vi "MBFL_Controller.vi"(0 "K":dbl[](array[numeric]), 1 "q_ref":dbl[](array[numeric]), 2 "q1":dbl, 3 "q2":dbl, 4 "q3":dbl, 5 "q4":dbl, 7 "K1":dbl, 9 "K2":dbl, 11 "K3":dbl, 13 "K4":dbl) -> (16 "u_out":dbl)   [LabVIEW 2021]
uses:
  <vilib>/Analysis/baseanly.llb/Real A x B.vi
  <vilib>/Analysis/Matrix/Numeric/Conversions/Matrix To Array - RM.vi
  <vilib>/Analysis/Matrix/Numeric/Conversions/Array To Matrix - RA2.vi
  <vilib>/Analysis/Matrix/Numeric/Multiply/Multiply - RM,R.vi
  <vilib>/Analysis/Matrix/NI_Matrix.lvlib
  <vilib>/Analysis/NI_AALBase.lvlib
panel:
  out "Etta(q)":dbl(graph)
  out "q1":dbl(graph)
  out "v(q)":dbl(graph)
  out "Control input u":dbl(graph)
  out "Gamma(q)":dbl(graph)
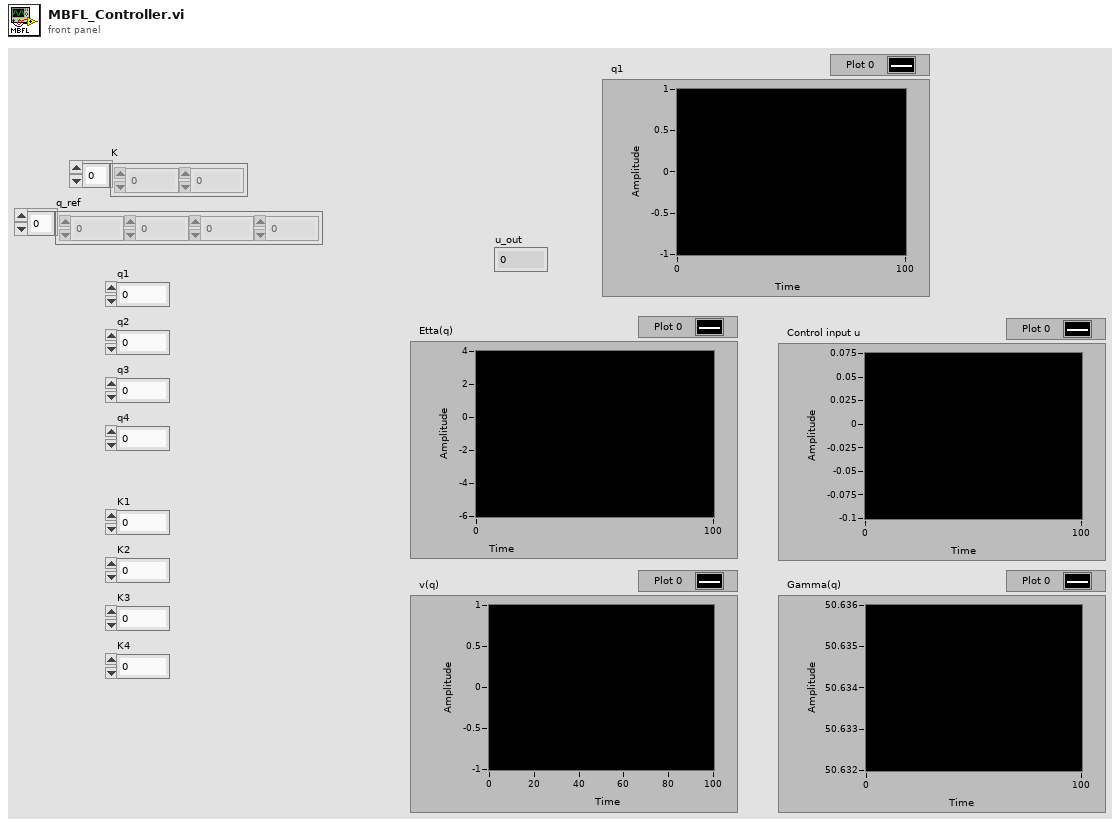
[diagram p1: front panel]
types:
  T1 = typedef "NI_Matrix.lvlib/RealMatrix.ctl" = dbl[][]
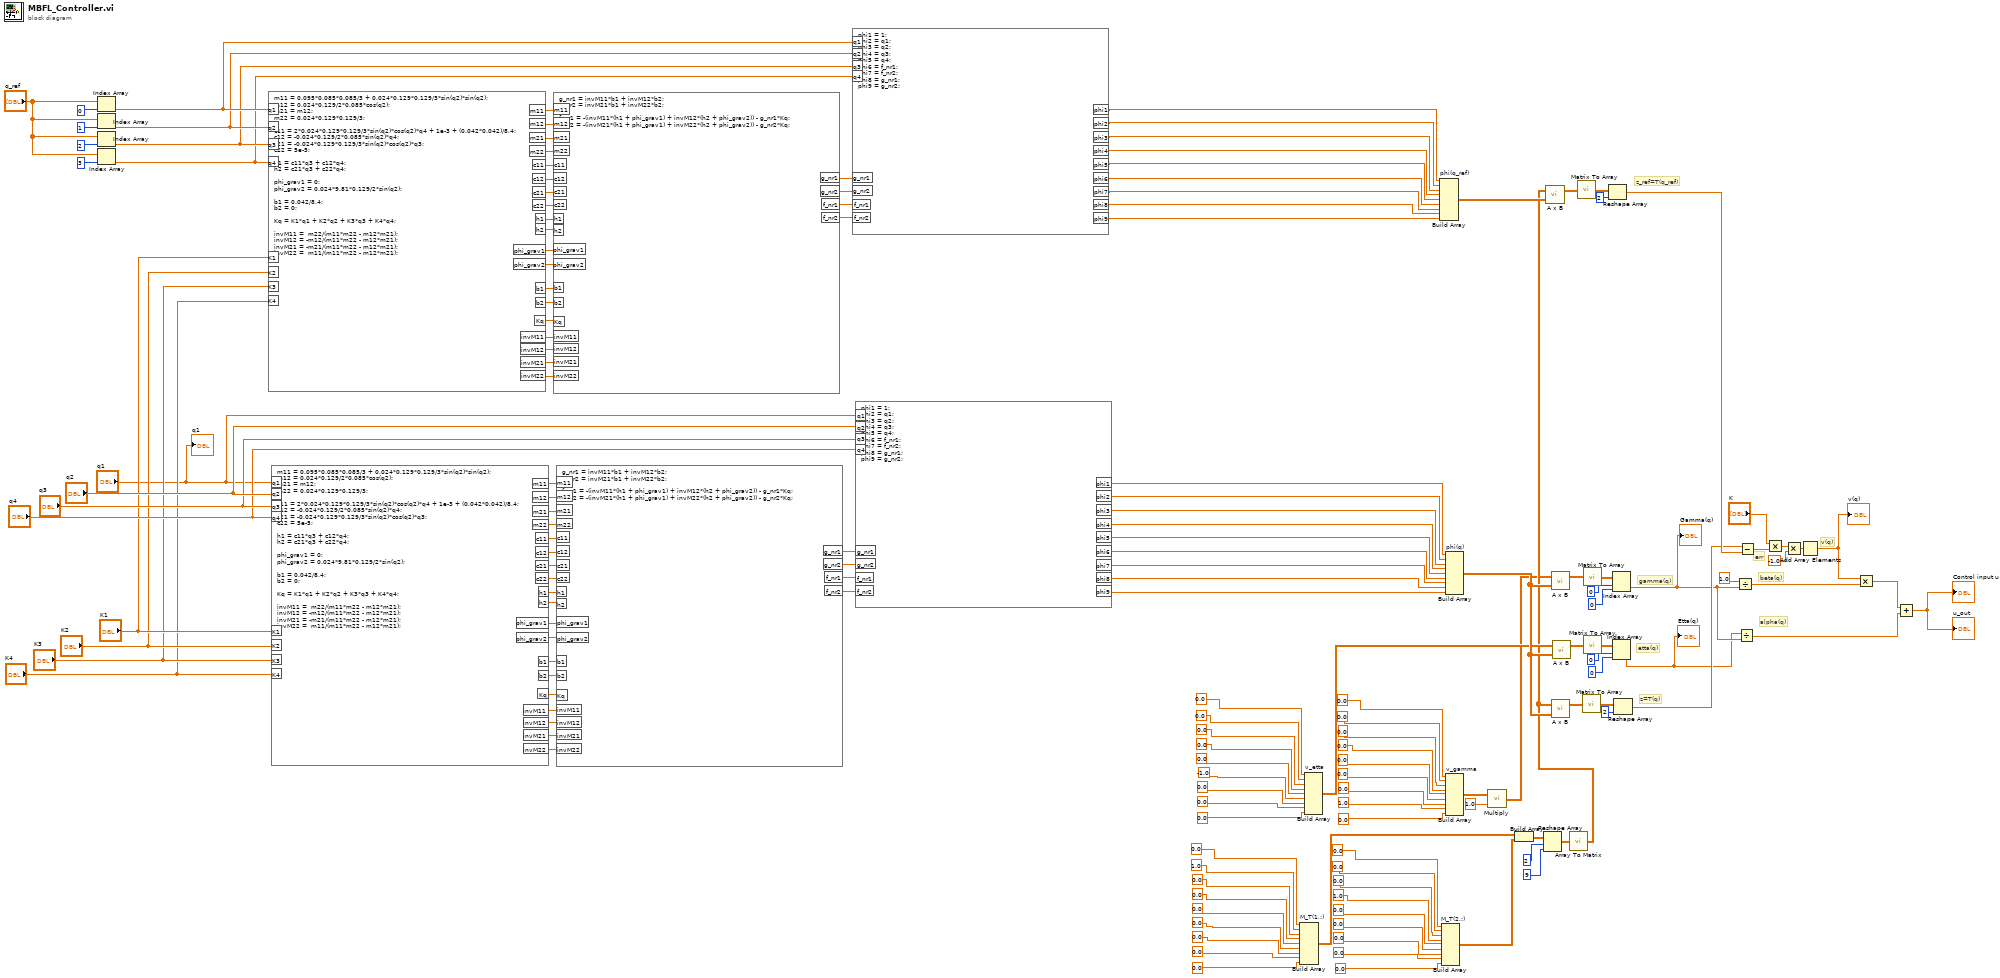
[diagram p0: block diagram]
diagram:
  # "alpha(q)"
  # "beta(q)"
  # "z_ref=T(q_ref)"
  # "v(q)"
  # "err"
  # "z=T(q)"
  # "etta(q)"
  # "gamma(q)"
  n1 = Index Array(array="q_ref", index=0 ("index 3")) -> (element=w29:dbl)
  n2 = Index Array(array="q_ref", index=1 ("index 4")) -> (element=w27:dbl)
  n3 = Index Array(array="q_ref", index=2 ("index 3")) -> (element=w26:dbl)
  n4 = Index Array(array="q_ref", index=3 ("index 4")) -> (element=w25:dbl)
  n5 = formula code="m11 = 0.095*0.085*0.085/3 + 0.024*0.129*0.129/3*sin(q2)*sin(q2);\nm12 = 0.024*0.129/2*0.085*cos(q2);\nm21 = m12;\nm22 = 0.024*0.129*0.129/3;\n\nc11 = 2*0.024*0.129*0.129/3*sin(q2)*cos(q2)*q4 + 1e-3 + (0.042*0.042)/8.4;\nc12 = -0.024*0.129/2*0.085*sin(q2)*q4;\nc21 = -0.024*0.129*0.129/3*sin(q2)*cos(q2)*q3;\nc22 = 5e-5;\n\nh1 = c11*q3 + c12*q4;\nh2 = c21*q3 + c22*q4;\n\nphi_grav1 = 0;\nphi_grav2 = 0.024*9.81*0.129/2*sin(q2);\n\nb1 = 0.042/8.4;\nb2 = 0;\n\nKq = K1*q1 + K2*q2 + K3*q3 + K4*q4;\n\ninvM11 =  m22/(m11*m22 - m12*m21);\ninvM12 = -m12/(m11*m22 - m12*m21);\ninvM21 = -m21/(m11*m22 - m12*m21);\ninvM22 =  m11/(m11*m22 - m12*m21);"("q1"=w29, "q2"=w27, "q3"=w26, "q4"=w25, "K1"="K1", "K2"="K2", "K3"="K3", "K4"="K4") -> ("m11"=w70:dbl, "m12"=w69:dbl, "m21"=w68:dbl, "m22"=w67:dbl, "c11"=w66:dbl, "c12"=w65:dbl, "c21"=w64:dbl, "c22"=w63:dbl, "h1"=w62:dbl, "h2"=w61:dbl, "phi_grav1"=w60:dbl, "phi_grav2"=w59:dbl, "b1"=w58:dbl, "b2"=w57:dbl, "Kq"=w56:dbl, "invM11"=w55:dbl, "invM12"=w54:dbl, "invM21"=w53:dbl, "invM22"=w52:dbl)
  n6 = formula code="m11 = 0.095*0.085*0.085/3 + 0.024*0.129*0.129/3*sin(q2)*sin(q2);\nm12 = 0.024*0.129/2*0.085*cos(q2);\nm21 = m12;\nm22 = 0.024*0.129*0.129/3;\n\nc11 = 2*0.024*0.129*0.129/3*sin(q2)*cos(q2)*q4 + 1e-3 + (0.042*0.042)/8.4;\nc12 = -0.024*0.129/2*0.085*sin(q2)*q4;\nc21 = -0.024*0.129*0.129/3*sin(q2)*cos(q2)*q3;\nc22 = 5e-5;\n\nh1 = c11*q3 + c12*q4;\nh2 = c21*q3 + c22*q4;\n\nphi_grav1 = 0;\nphi_grav2 = 0.024*9.81*0.129/2*sin(q2);\n\nb1 = 0.042/8.4;\nb2 = 0;\n\nKq = K1*q1 + K2*q2 + K3*q3 + K4*q4;\n\ninvM11 =  m22/(m11*m22 - m12*m21);\ninvM12 = -m12/(m11*m22 - m12*m21);\ninvM21 = -m21/(m11*m22 - m12*m21);\ninvM22 =  m11/(m11*m22 - m12*m21);"("q1"="q1", "q2"="q2", "q3"="q3", "q4"="q4", "K1"="K1", "K2"="K2", "K3"="K3", "K4"="K4") -> ("m11"=w96:dbl, "m12"=w95:dbl, "m21"=w94:dbl, "m22"=w93:dbl, "c11"=w92:dbl, "c12"=w91:dbl, "c21"=w90:dbl, "c22"=w89:dbl, "h1"=w88:dbl, "h2"=w87:dbl, "phi_grav1"=w86:dbl, "phi_grav2"=w85:dbl, "b1"=w84:dbl, "b2"=w83:dbl, "Kq"=w82:dbl, "invM11"=w81:dbl, "invM12"=w80:dbl, "invM21"=w79:dbl, "invM22"=w78:dbl)
  n7 = formula code="g_nr1 = invM11*b1 + invM12*b2;\ng_nr2 = invM21*b1 + invM22*b2;\n\nf_nr1 = -(invM11*(h1 + phi_grav1) + invM12*(h2 + phi_grav2)) - g_nr1*Kq;\nf_nr2 = -(invM21*(h1 + phi_grav1) + invM22*(h2 + phi_grav2)) - g_nr2*Kq;"("m11"=w70, "m12"=w69, "m21"=w68, "m22"=w67, "invM11"=w55, "invM12"=w54, "invM21"=w53, "invM22"=w52, "c11"=w66, "c12"=w65, "c21"=w64, "c22"=w63, "h1"=w62, "h2"=w61, "phi_grav1"=w60, "phi_grav2"=w59, "b1"=w58, "b2"=w57, "Kq"=w56) -> ("g_nr1"=w51:dbl, "g_nr2"=w50:dbl, "f_nr1"=w49:dbl, "f_nr2"=w48:dbl)
  n8 = formula code="g_nr1 = invM11*b1 + invM12*b2;\ng_nr2 = invM21*b1 + invM22*b2;\n\nf_nr1 = -(invM11*(h1 + phi_grav1) + invM12*(h2 + phi_grav2)) - g_nr1*Kq;\nf_nr2 = -(invM21*(h1 + phi_grav1) + invM22*(h2 + phi_grav2)) - g_nr2*Kq;"("m11"=w96, "m12"=w95, "m21"=w94, "m22"=w93, "invM11"=w81, "invM12"=w80, "invM21"=w79, "invM22"=w78, "c11"=w92, "c12"=w91, "c21"=w90, "c22"=w89, "h1"=w88, "h2"=w87, "phi_grav1"=w86, "phi_grav2"=w85, "b1"=w84, "b2"=w83, "Kq"=w82) -> ("g_nr1"=w77:dbl, "g_nr2"=w76:dbl, "f_nr1"=w75:dbl, "f_nr2"=w74:dbl)
  n9 = formula code="phi1 = 1;\nphi2 = q1;\nphi3 = q2;\nphi4 = q3;\nphi5 = q4;\nphi6 = f_nr1;\nphi7 = f_nr2;\nphi8 = g_nr1;\nphi9 = g_nr2;"("q1"=w29, "q2"=w27, "q3"=w26, "q4"=w25, "g_nr1"=w51, "g_nr2"=w50, "f_nr1"=w49, "f_nr2"=w48) -> ("phi1"=w47:dbl, "phi2"=w46:dbl, "phi3"=w45:dbl, "phi4"=w44:dbl, "phi5"=w43:dbl, "phi6"=w42:dbl, "phi7"=w41:dbl, "phi8"=w40:dbl, "phi9"=w39:dbl)
  n10 = formula code="phi1 = 1;\nphi2 = q1;\nphi3 = q2;\nphi4 = q3;\nphi5 = q4;\nphi6 = f_nr1;\nphi7 = f_nr2;\nphi8 = g_nr1;\nphi9 = g_nr2;"("q1"="q1", "q2"="q2", "q3"="q3", "q4"="q4", "g_nr1"=w77, "g_nr2"=w76, "f_nr1"=w75, "f_nr2"=w74) -> ("phi1"=w105:dbl, "phi2"=w104:dbl, "phi3"=w103:dbl, "phi4"=w102:dbl, "phi5"=w101:dbl, "phi6"=w100:dbl, "phi7"=w99:dbl, "phi8"=w98:dbl, "phi9"=w97:dbl)
  n11 = Build Array "M_T(1,:)"(0.0, 1.0, 0.0, 0.0, 0.0, 0.0, 0.0, 0.0, 0.0) -> (w111:T1)
  n12 = Build Array "v_etta"(0.0, 0.0, 0.0, 0.0, 0.0, -1.0, 0.0, 0.0, 0.0) -> (w150:T1)
  n13 = Build Array "phi(q_ref)"(w47, w46, w45, w44, w43, w42, w41, w40, w39) -> (w35:T1)
  n14 = Build Array "M_T(2,:)"(0.0, 0.0, 0.0, 1.0, 0.0, 0.0, 0.0, 0.0, 0.0) -> (w110:T1)
  n15 = Build Array "phi(q)"(w105, w104, w103, w102, w101, w100, w99, w98, w97) -> (w151:T1)
  n16 = Build Array "v_gamma"(0.0, 0.0, 0.0, 0.0, 0.0, 0.0, 0.0, 1.0, 0.0) -> (w15:T1)
  n17 = call-poly <vilib>:"Multiply.vi"("Real Scalar c"=1.0, "Real Matrix A"=w15) -> ("A * c"=w17:T1)
  n18 = Build Array(w111, w110) -> (w109:dbl[][][])
  n19 = Reshape Array(w109, 2, 9) -> (w106:dbl[][])
  n20 = call-poly <vilib>:"A x B.vi"("B"=w151, "A"=w17) -> ("A x B"=w146:T1)  [unwired: 1 out]
  n21 = call-poly <vilib>:"A x B.vi"("B"=w151, "A"=w150) -> ("A x B"=w141:T1)  [unwired: 1 out]
  n22 = call-poly <vilib>:"Array To Matrix.vi"("Real 2D Array"=w106) -> ("Real Matrix"=w34:T1)
  n23 = call-poly <vilib>:"A x B.vi"("B"=w35, "A"=w34) -> ("A x B"=w38:T1)  [unwired: 1 out]
  n24 = call-poly <vilib>:"A x B.vi"("B"=w151, "A"=w34) -> ("A x B"=w142:T1)  [unwired: 1 out]
  n25 = call-poly <vilib>:"Matrix To Array.vi"("Real Matrix"=w38) -> ("Real 2D Array"=w37:dbl[][])
  n26 = call-poly <vilib>:"Matrix To Array.vi"("Real Matrix"=w142) -> ("Real 2D Array"=w140:dbl[][])
  n27 = call-poly <vilib>:"Matrix To Array.vi"("Real Matrix"=w146) -> ("Real 2D Array"=w149:dbl[][])
  n28 = call-poly <vilib>:"Matrix To Array.vi"("Real Matrix"=w141) -> ("Real 2D Array"=w145:dbl[][])
  n29 = Reshape Array(w37, 2 ("dimension size")) -> (w12:dbl[])
  n30 = Index Array ("Index Array 2")(array=w149, index (row)=0 ("index 3"), index (col)=0 ("index 4")) -> (element=w7:dbl)
  "Gamma(q)" <- w7
  n31 = Index Array ("Index Array 2")(array=w145, index (row)=0 ("index 3"), index (col)=0 ("index 4")) -> (element=w6:dbl)
  "Etta(q)" <- w6
  n32 = Reshape Array(w140, 2 ("dimension size")) -> (w11:dbl[])
  n33 = Divide(x=1.0, y=w7) -> (x/y=w4:dbl)
  n34 = Divide(x=w6, y=w7) -> (x/y=w2:dbl)
  n35 = Subtract(x=w11, y=w12) -> (x-y=w137:dbl[])
  n36 = Multiply(x="K", y=w137) -> (x*y=w10:dbl[])
  n37 = Multiply(x=w10, y=-1.0) -> (x*y=w9:dbl[])
  n38 = Add Array Elements(numeric array=w9) -> (sum=w5:dbl)
  "v(q)" <- w5
  n39 = Multiply(x=w5, y=w4) -> (x*y=w3:dbl)
  n40 = Add(x=w3, y=w2) -> (x+y=→"u_out" →"Control input u":dbl)
  "q1" <- "q1"
